vi "CallDLL.vi"() -> ()   [LabVIEW 2013]
uses:
  reconrepo/imagereconstruction/x64/Debug/labviewdll.dll
panel:
  in  "Dummy Value":sgl
  out "Average Value":sgl
  out "Error":i32
  in  "Array":dbl[](array[numeric])
  in  "Boolean":bool
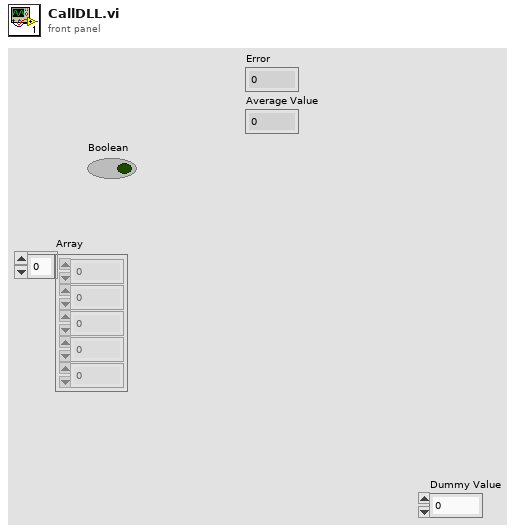
[diagram p1: front panel]
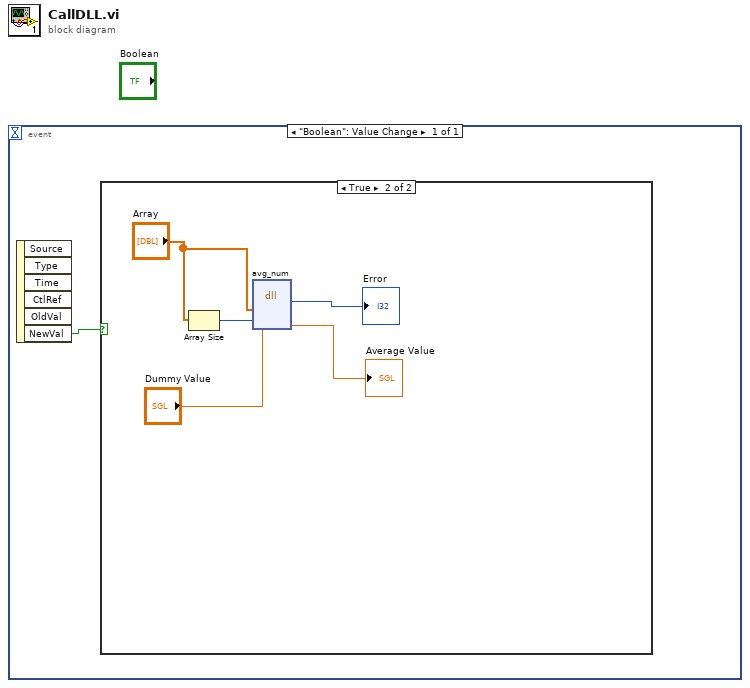
[diagram p0: block diagram]
diagram:
  n1 = event shown="[0] \"Boolean\": Value Change" {
    selector: _ -> [_]
    dyn-events: _ -> [_]
    timeout: _ -> [_]
    event "Boolean": Value Change {
      n2 = event-data() -> ("NewVal"=w1:bool)  [unwired: 1 in, 5 out]
      n3 = case shown="True" w1 {
        frame False {
        }
        frame True {
          n4 = Array Size(array="Array") -> (size(s)=w6:i32)
          n5 = dll-call lib="D:/work/uni/FYP/reconrepo/imagereconstruction/x64/Debug/labviewdll.dll" fn="avg_num"("a"="Array", "size"=w6, "avg"="Dummy Value") -> ("return type"=→"Error":i32, "avg"=→"Average Value":sgl)  [unwired: 5 in, 2 out]
        }
      }
    }
  }
